vi "G#Object_Open.vi"(0 "reference in":refnum<class "G#SubClass1.lvclass">, 5 "error in (no error)":errorcluster) -> (14 "reference out":refnum<class "G#SubClass1.lvclass">, 19 "error out":errorcluster)   [LabVIEW 2020, in "G#SubClass1.lvclass"]
uses:
  G#SubClass1.lvclass
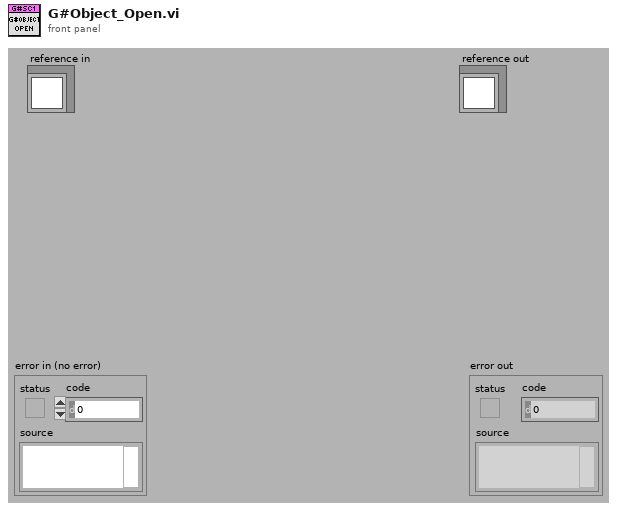
[diagram p1: front panel]
types:
  T1 = typedef "G#SubClass1.lvclass/ObjectAttributesRef.ctl" = refnum<data-value>
  T2 = typedef "G#SubClass1.lvclass/ObjectAttributes.ctl" = cluster{"SubNumeric":dbl, "TestQueue":refnum<queue>}
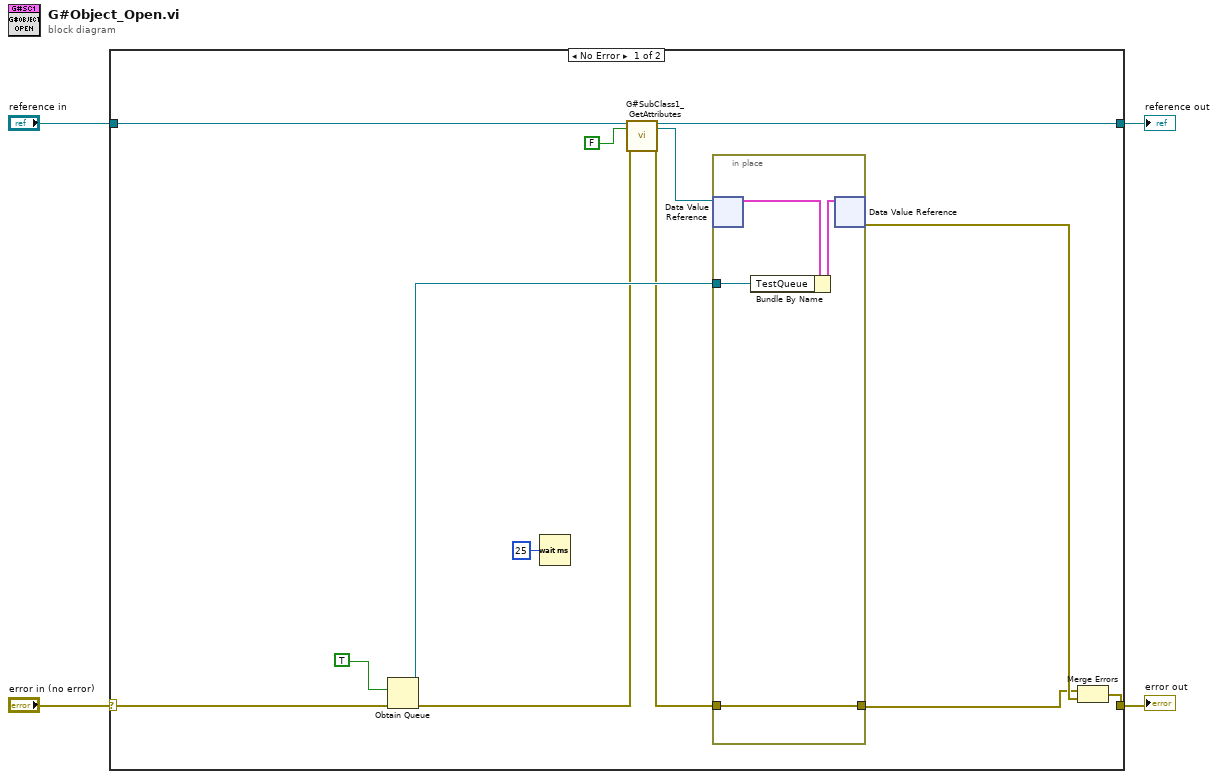
[diagram p0: block diagram]
diagram:
  n1 = case shown="No Error" "error in (no error)" {
    selector: "error in (no error)" -> [w13 w23]
    tunnel: [w17 w23] -> w3
    tunnel: [w9 w22] -> w1
    tunnel: "reference in" -> [w10 w22]
    frame No Error {
      n2 = Obtain Queue(element data type=TRUE, error in (no error)=w13) -> (queue out=w12:refnum<queue>, error out=w8:errorcluster)  [unwired: 3 in, 1 out]
      n3 = Wait (ms)(milliseconds to wait=u32 25) -> ()  [unwired: 1 out]
      n4 = call "G#SubClass1_GetAttributes.vi"("reference in"=w10, "return data? (T)"=FALSE, "error in (no error)"=w8) -> ("reference out"=w9:refnum<class "G#SubClass1.lvclass">, "attributes ref"=w5:T1, "error out"=w7:errorcluster)  [unwired: 13 in, 1 out]
      n5 = in-place {
        in-place-border: w7 -> [w21]
        in-place-border: [w21] -> w15
        in-place-border: w12 -> [w18]
        n6 = in-place-dvr #1(w5) -> (w20:T2)  [unwired: 1 out]
        n7 = Bundle By Name(cluster=w20, "TestQueue"=w18) -> (w19:T2)
        n8 = in-place-dvr #1(w19) -> (w16:errorcluster)  [unwired: 1 out]
      }
      n9 = Merge Errors(w15, w16) -> (w17:errorcluster)
    }
    frame Error {
    }
  }
  "error out" <- w3
  "reference out" <- w1
